vi "Counter.vi"() -> ()   [LabVIEW 2017]
uses:
  <vilib>/addons/database/Connection.llb/DB Tools Open Connec (String).vi
  Global/Global 1.vi
  <vilib>/addons/database/NI_Database_API.lvlib
panel:
  in  "Reset Square":bool
  in  "RECIPE NAME":string
  out "RUNNING LOADED RECIPE":string
  in  "BARCODE RECIPE":string(combo)
  in  "Delete Square":bool
  in  "Save Square":bool
  in  "OK2":bool
  in  "FROM":timestamp format="%<%x>T"
  out "error out":errorcluster
  in  "error in (no error)":errorcluster
  in  "EXIT":bool
  in  "SHIFT":string(combo)
  in  "TO":timestamp format="%<%x>T"
  out "OK":i32
  out "TOTAL":i32
  out "NOK":i32
  # "COUNTER"
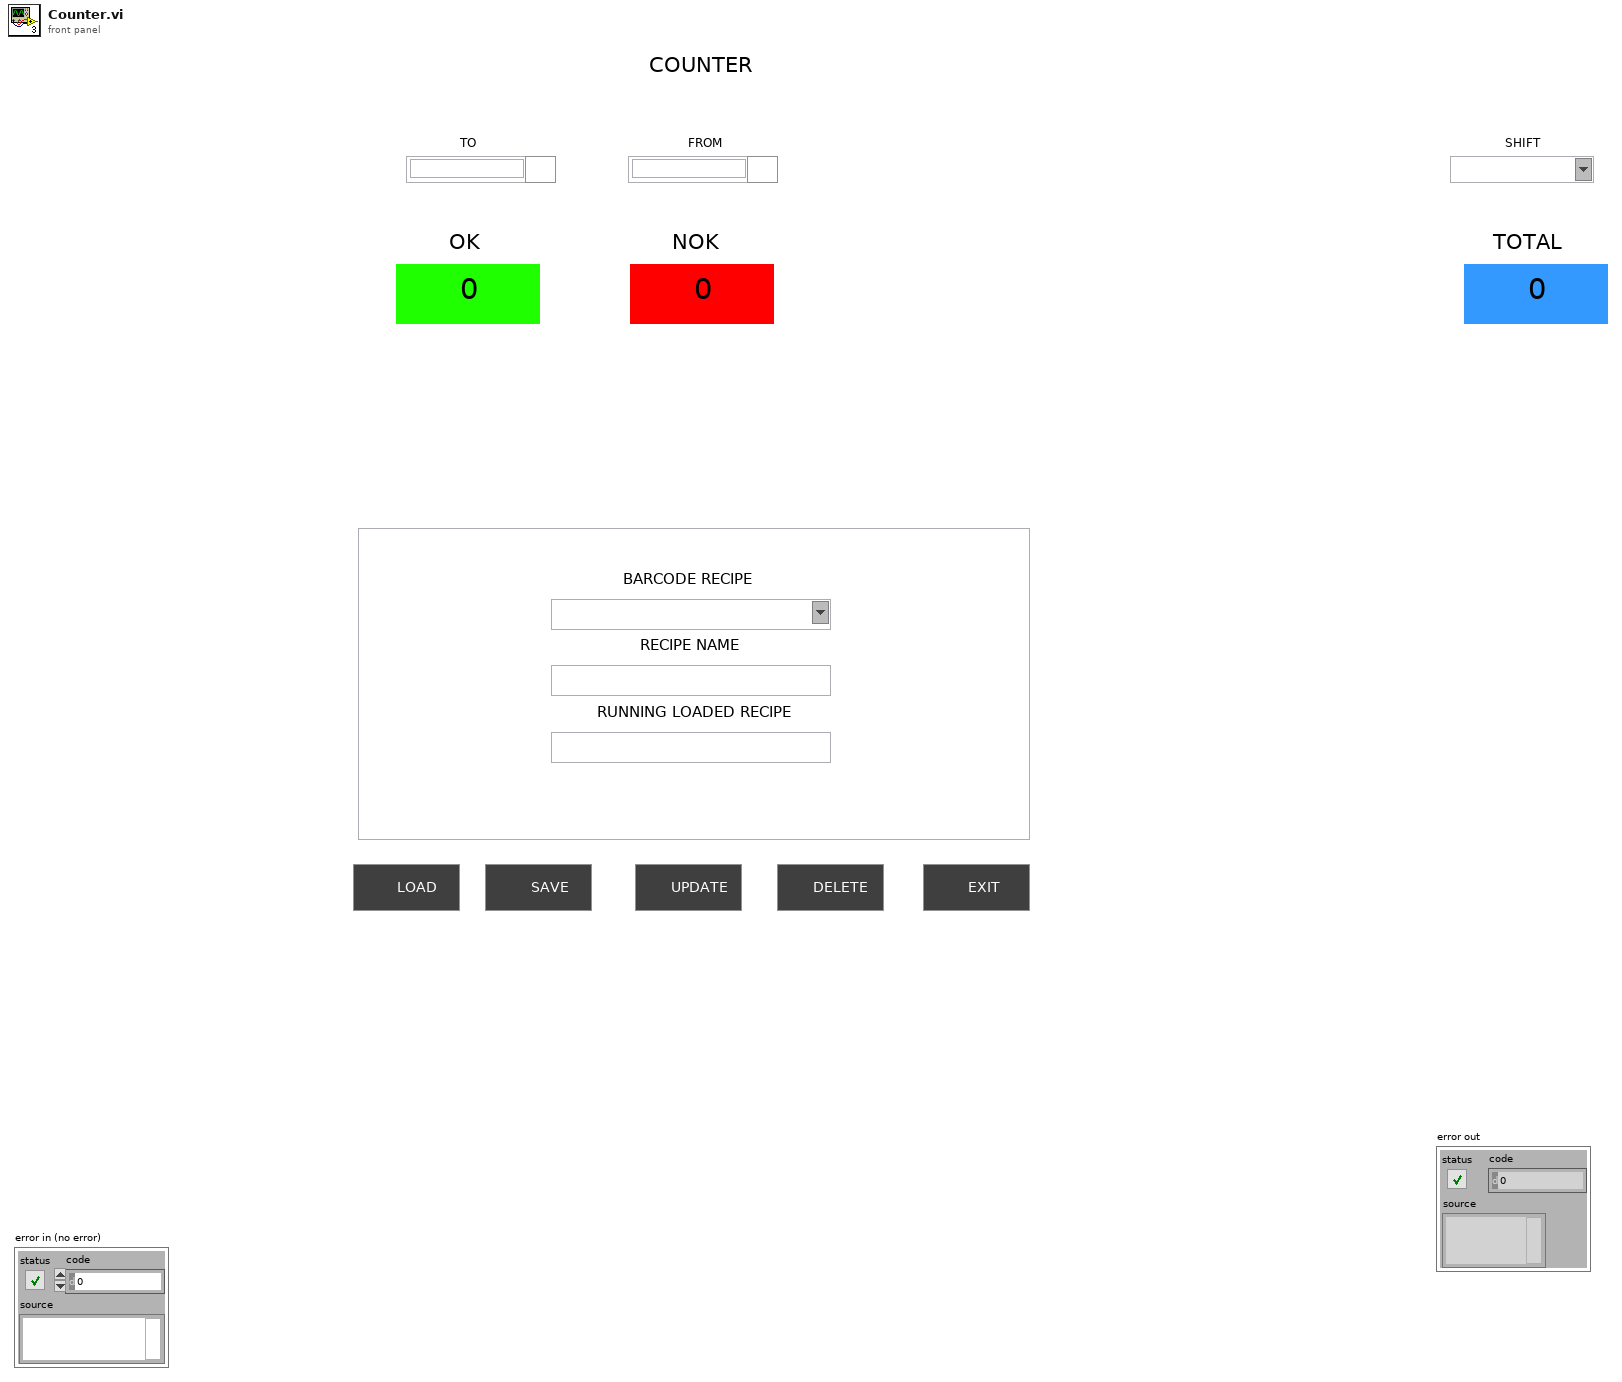
[diagram p1: front panel]
types:
  T1 = typedef "NI_Database_API.lvlib/Conn ObjectReference.ctl" = refnum<k1>
  T2 = cluster{" BARCODE RECIPE":string, "RECIPE NAME":string}
  T3 = enum32{"invalid app kind", "Development System", "Run Time System", "Student Edition", "Embedded LabVIEW", "Evaluation", "Custom"}
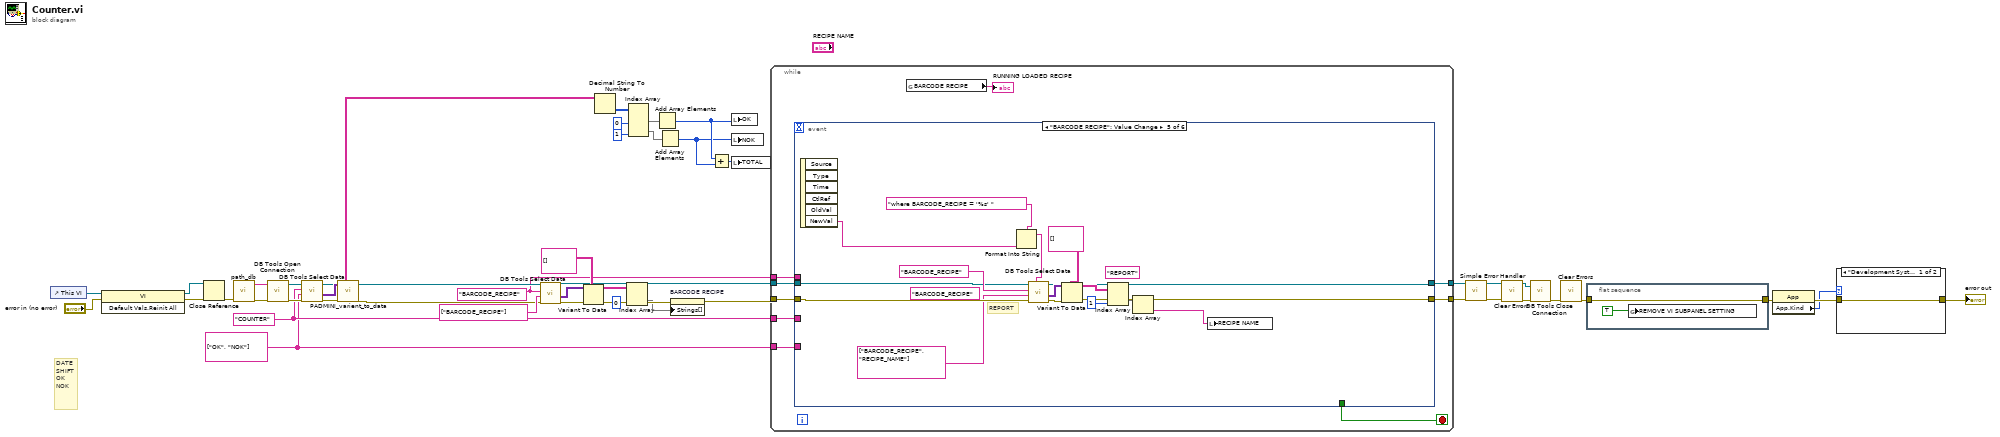
[diagram p0: block diagram]
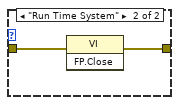
[diagram p2: hidden frame]
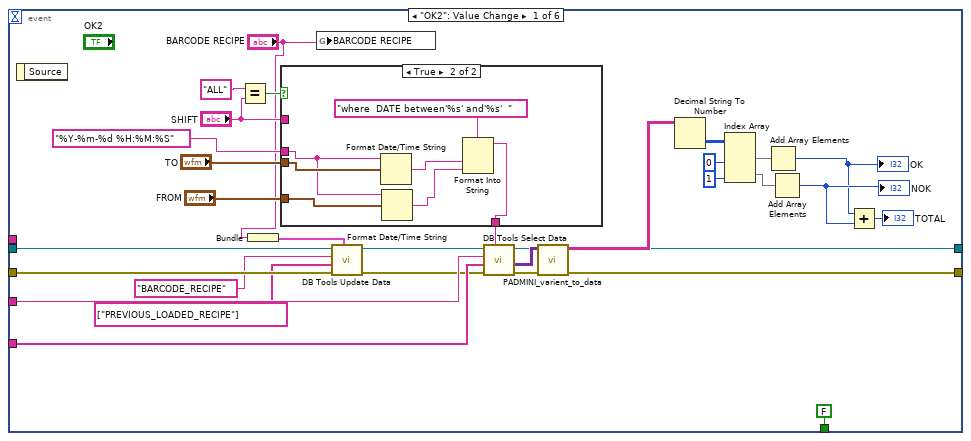
[diagram p3: hidden frame]
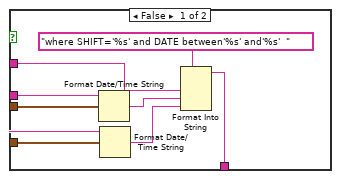
[diagram p4: hidden frame]
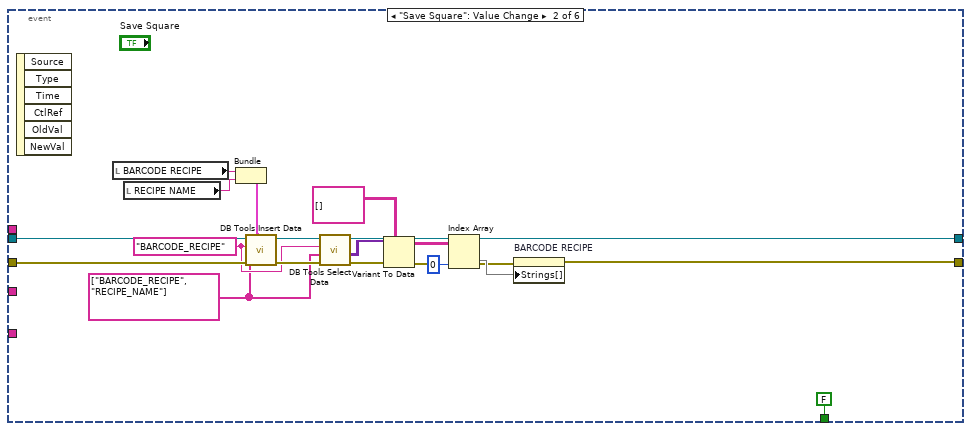
[diagram p5: hidden frame]
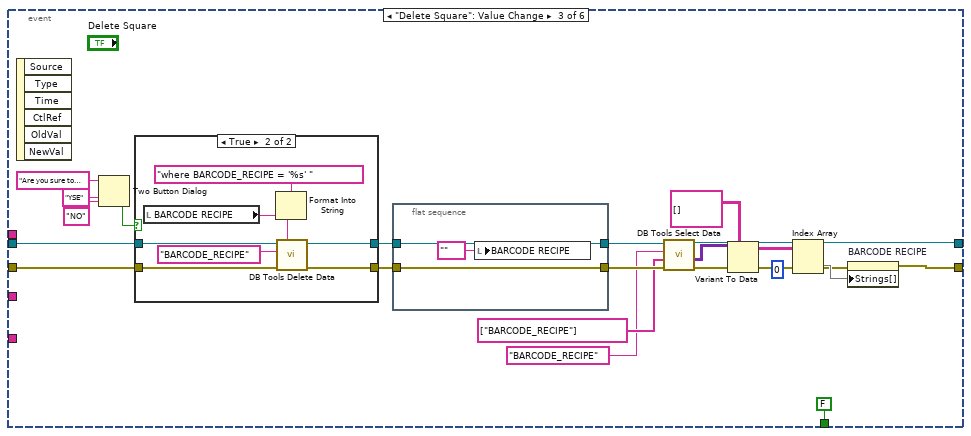
[diagram p6: hidden frame]
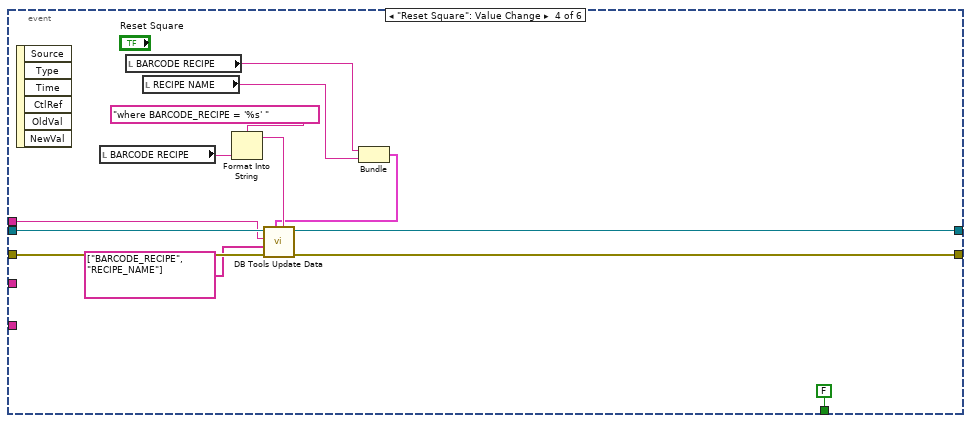
[diagram p8: hidden frame]
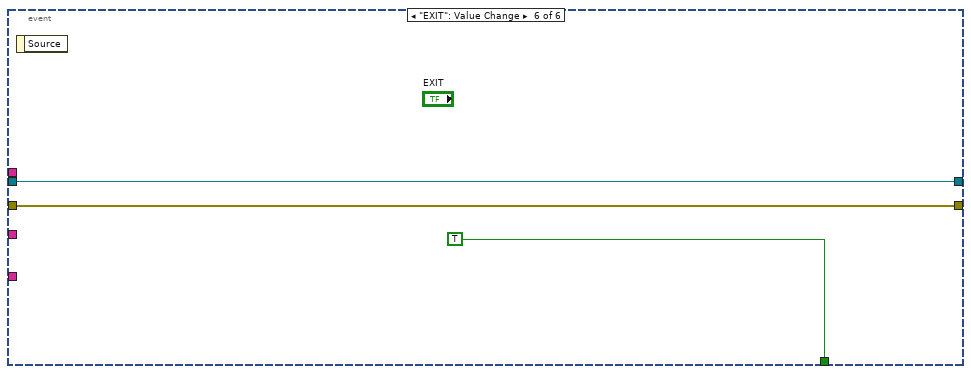
[diagram p9: hidden frame]
diagram:
  w1 = "BARCODE_RECIPE" ("table")
  w14 = string[] ["OK", "NOK"]
  w15 = "COUNTER"
  # "DATE\nSHIFT\nOK\nNOK"
  n1 = control-ref of="This VI"() -> (w43:refnum<vi>)
  n2 = invoke class="VI" method="Default Vals.Reinit All"(reference=w43, error in="error in (no error)") -> (reference out=w41:refnum<vi>, error out=w40:errorcluster)  [unwired: 1 in, 1 out]
  n3 = Close Reference(reference=w41, error in (no error)=w40) -> (error out=w39:errorcluster)
  n4 = call "path_db.vi"("error in"=w39) -> ("error out"=w45:errorcluster, "resulting string"=w44:string)  [unwired: 9 in]
  n5 = call-poly <vilib>:"DB Tools Open Connection.vi"("error in (no error)"=w45, "connection information"=w44) -> ("error out"=w26:errorcluster, "connection reference"=w38:T1)  [unwired: 6 in]
  n6 = call <vilib>:"DB Tools Select Data.vi"("error in (no error)"=w26, "columns"=w14, "table"=w15, "connection reference"=w38) -> ("error out"=w25:errorcluster, "data"=w27:variant[][], "connection reference out"=w4:T1)  [unwired: 2 in]
  n7 = call "PADMINI_varient_to_data.vi"("error in (no error)"=w25, "data"=w27) -> ("error out"=w2:errorcluster, "Array"=w24:string[][])  [unwired: 8 in]
  n8 = call <vilib>:"DB Tools Select Data.vi"("error in (no error)"=w2, "columns"=string[] ["BARCODE_RECIPE"], "table"=w1, "connection reference"=w4) -> ("error out"=w11:errorcluster, "data"=w7:variant[][], "connection reference out"=w5:T1)  [unwired: 2 in]
  n9 = Variant To Data(error in=w11, type=string[][] [], Variant=w7) -> (data=w6:string[][], error out=w13:errorcluster)
  n10 = Decimal String To Number(string=w24) -> (number=w23:i32[][])  [unwired: 2 in, 1 out]
  n11 = Index Array(array=w6, index (col)=0 ("disabled index (col)")) -> (element=w9:string[])  [unwired: 1 in]
  n12 = Index Array(array=w23, index (col) #1=0 ("disabled index (col)"), index (col) #2=1 ("index (col)")) -> (element #1=w20:i32[], element #2=w19:i32[])  [unwired: 2 in]
  n13 = Add Array Elements(numeric array=w20) -> (sum=w18:i32)
  n14 = Add Array Elements(numeric array=w19) -> (sum=w17:i32)
  n15 = property on="BARCODE RECIPE" class="CmbBox"(error in=w13, "Strings[]"=w9) -> (error out=w10:errorcluster)  [unwired: 1 in, 1 out]
  n16 = Add(x=w18, y=w17) -> (x+y=w16:i32)
  n17 = local write "OK"(w18) -> ()
  n18 = local write "NOK"(w17) -> ()
  n19 = local write "TOTAL"(w16) -> ()
  n20 = while {
    tunnel: w10 -> [w53]
    tunnel: w5 -> [w52]
    tunnel: [w51] -> w29
    tunnel: [w50] -> w28
    tunnel: w15 -> [w49]
    tunnel: w14 -> [w48]
    tunnel: w1 -> [w46]
    stop <- w54 stop-if-true
    n21 = event shown="[4] \"BARCODE RECIPE\": Value Change" {
      selector: _ -> [_ _ _ _ _ _]
      dyn-events: _ -> [_ _ _ _ _ _]
      timeout: _ -> [_ _ _ _ _ _]
      tunnel: [FALSE FALSE FALSE FALSE _ TRUE] -> w54
      tunnel: w53 -> [w60 w119 w140 w166 w176 w184]
      tunnel: w52 -> [w62 w118 w141 w167 w177 w185]
      tunnel: [w76 w111 w128 w165 w170 w185] -> w51
      tunnel: [w77 w104 w127 w164 w169 w184] -> w50
      tunnel: w49 -> [w75 _ _ _ _ _]
      tunnel: w48 -> [w74 _ _ _ _ _]
      tunnel: w46 -> [_ _ _ w163 _ _]
      event "OK2": Value Change {
        n22 = event-data() -> ()  [unwired: 1 in, 1 out]
        n23 = Equal?(x="ALL", y="SHIFT") -> (x = y?=w65:bool)
        n24 = Bundle("BARCODE RECIPE"="BARCODE RECIPE") -> (w55:cluster{" BARCODE RECIPE":string})  [unwired: 1 in]
        n25 = case shown="True" w65 {
          tunnel: [w93 w95] -> w70
          tunnel: "SHIFT" -> [w91 _]
          tunnel: "TO" -> [w90 w99]
          tunnel: "FROM" -> [w88 w97]
          tunnel: "%Y-%m-%d %H:%M:%S" ("time format string (%c)") -> [w86 w98]
          frame False {
            n26 = Format Date/Time String(time format string (%c)=w86, seconds (now)=w90) -> (date/time string=w89:string)  [unwired: 1 in]
            n27 = Format Date/Time String(time format string (%c)=w86, seconds (now)=w88) -> (date/time string=w87:string)  [unwired: 1 in]
            n28 = Format Into String(format string="where SHIFT='%s' and DATE between'%s' and'%s'  ", w91, w89, w87) -> (resulting string=w93:string)  [unwired: 2 in, 1 out]
          }
          frame True {
            n29 = Format Date/Time String(time format string (%c)=w98, seconds (now)=w99) -> (date/time string=w100:string)  [unwired: 1 in]
            n30 = Format Date/Time String(time format string (%c)=w98, seconds (now)=w97) -> (date/time string=w96:string)  [unwired: 1 in]
            n31 = Format Into String(format string="where  DATE between'%s' and'%s'  ", w100, w96) -> (resulting string=w95:string)  [unwired: 2 in, 1 out]
          }
        }
        n32 = global write "Global 1.vi" "BARCODE RECIPE"("BARCODE RECIPE") -> ()
        n33 = call <vilib>:"DB Tools Update Data.vi"("data"=w55, "error in (no error)"=w60, "columns"=string[] ["PREVIOUS_LOADED_RECIPE"], "table"="BARCODE_RECIPE", "connection reference"=w62) -> ("error out"=w59:errorcluster, "connection reference out"=w61:T1)  [unwired: 5 in]
        n34 = call <vilib>:"DB Tools Select Data.vi"("condition"=w70, "error in (no error)"=w59, "columns"=w74, "table"=w75, "connection reference"=w61) -> ("error out"=w78:errorcluster, "data"=w85:variant[][], "connection reference out"=w76:T1)  [unwired: 1 in]
        n35 = call "PADMINI_varient_to_data.vi"("error in (no error)"=w78, "data"=w85) -> ("error out"=w77:errorcluster, "Array"=w84:string[][])  [unwired: 8 in]
        n36 = Decimal String To Number(string=w84) -> (number=w83:i32[][])  [unwired: 2 in, 1 out]
        n37 = Index Array(array=w83, index (col) #1=0 ("disabled index (col)"), index (col) #2=1 ("index (col)")) -> (element #1=w80:i32[], element #2=w79:i32[])  [unwired: 2 in]
        n38 = Add Array Elements(numeric array=w80) -> (sum=w71:i32)
        "OK" <- w71
        n39 = Add Array Elements(numeric array=w79) -> (sum=w72:i32)
        "NOK" <- w72
        n40 = Add(x=w71, y=w72) -> (x+y=→"TOTAL":i32)
      }
      event "Save Square": Value Change {
        w102 = string[] ["BARCODE_RECIPE", "RECIPE_NAME"] ("columns")
        w103 = "BARCODE_RECIPE" ("table")
        n41 = event-data() -> ()  [unwired: 1 in, 6 out]
        n42 = local read "BARCODE RECIPE"() -> (w117:string)
        n43 = local read "RECIPE NAME"() -> (w101:string)
        n44 = Bundle("BARCODE RECIPE"=w117, "RECIPE NAME"=w101) -> (w116:T2)  [unwired: 1 in]
        n45 = call <vilib>:"DB Tools Insert Data.vi"("data"=w116, "error in (no error)"=w119, "columns"=w102, "table"=w103, "connection reference"=w118) -> ("error out"=w114:errorcluster, "connection reference out"=w112:T1)  [unwired: 5 in]
        n46 = call <vilib>:"DB Tools Select Data.vi"("error in (no error)"=w114, "columns"=w102, "table"=w103, "connection reference"=w112) -> ("error out"=w113:errorcluster, "data"=w109:variant[][], "connection reference out"=w111:T1)  [unwired: 2 in]
        n47 = Variant To Data(error in=w113, type=string[][] [], Variant=w109) -> (data=w108:string[][], error out=w105:errorcluster)
        n48 = Index Array(array=w108, index (col)=0 ("disabled index (col)")) -> (element=w106:string[])  [unwired: 1 in]
        n49 = property on="BARCODE RECIPE" class="CmbBox"(error in=w105, "Strings[]"=w106) -> (error out=w104:errorcluster)  [unwired: 1 in, 1 out]
      }
      event "Delete Square": Value Change {
        n50 = event-data() -> ()  [unwired: 1 in, 6 out]
        n51 = Two Button Dialog(message="Are you sure to want delete this barcode recipe?", 1:"NO" ("F button name (\"Cancel\")"), 2:"YSE" ("T button name (\"OK\")")) -> (T button?=w121:bool)
        n52 = case shown="True" w121 {
          tunnel: w141 -> [w143 w151]
          tunnel: w140 -> [w142 w150]
          tunnel: [w142 w146] -> w139
          tunnel: [w143 w145] -> w138
          frame False {
          }
          frame True {
            n53 = local read "BARCODE RECIPE"() -> (w148:string)
            n54 = Format Into String(format string="where BARCODE_RECIPE = '%s' ", w148) -> (resulting string=w147:string)  [unwired: 2 in, 1 out]
            n55 = call <vilib>:"DB Tools Delete Data.vi"("condition"=w147, "error in (no error)"=w150, "table"="BARCODE_RECIPE", "connection reference"=w151) -> ("error out"=w146:errorcluster, "connection reference out"=w145:T1)  [unwired: 6 in]
          }
        }
        n56 = flat-sequence {
          tunnel: [w154] -> w129
          tunnel: w139 -> [w154]
          tunnel: [w152] -> w130
          tunnel: w138 -> [w152]
          frame #0 {
            n57 = local write "BARCODE RECIPE"("" ("BARCODE RECIPE")) -> ()
          }
        }
        n58 = call <vilib>:"DB Tools Select Data.vi"("error in (no error)"=w129, "columns"=string[] ["BARCODE_RECIPE"], "table"="BARCODE_RECIPE", "connection reference"=w130) -> ("error out"=w137:errorcluster, "data"=w136:variant[][], "connection reference out"=w128:T1)  [unwired: 2 in]
        n59 = Variant To Data(error in=w137, type=string[][] [], Variant=w136) -> (data=w135:string[][], error out=w133:errorcluster)
        n60 = Index Array(array=w135, index (col)=0 ("disabled index (col)")) -> (element=w134:string[])  [unwired: 1 in]
        n61 = property on="BARCODE RECIPE" class="CmbBox"(error in=w133, "Strings[]"=w134) -> (error out=w127:errorcluster)  [unwired: 1 in, 1 out]
      }
      event "Reset Square": Value Change {
        n62 = event-data() -> ()  [unwired: 1 in, 6 out]
        n63 = local read "BARCODE RECIPE"() -> (w161:string)
        n64 = local read "BARCODE RECIPE"() -> (w158:string)
        n65 = local read "RECIPE NAME"() -> (w157:string)
        n66 = Format Into String(format string="where BARCODE_RECIPE = '%s' ", w161) -> (resulting string=w159:string)  [unwired: 2 in, 1 out]
        n67 = Bundle("BARCODE RECIPE"=w158, "RECIPE NAME"=w157) -> (w156:T2)  [unwired: 1 in]
        n68 = call <vilib>:"DB Tools Update Data.vi"("condition"=w159, "data"=w156, "error in (no error)"=w166, "columns"=string[] ["BARCODE_RECIPE", "RECIPE_NAME"], "table"=w163, "connection reference"=w167) -> ("error out"=w164:errorcluster, "connection reference out"=w165:T1)  [unwired: 4 in]
      }
      event "BARCODE RECIPE": Value Change {
        (unwired) "BARCODE_RECIPE" ("String")
        (unwired) "REPORT"
        # "REPORT"
        n69 = event-data() -> ("NewVal"=w173:string)  [unwired: 1 in, 5 out]
        n70 = Format Into String(format string="where BARCODE_RECIPE = '%s' ", w173) -> (resulting string=w174:string)  [unwired: 2 in, 1 out]
        n71 = call <vilib>:"DB Tools Select Data.vi"("condition"=w174, "error in (no error)"=w176, "columns"=string[] ["BARCODE_RECIPE", "RECIPE_NAME"], "table"="BARCODE_RECIPE", "connection reference"=w177) -> ("error out"=w182:errorcluster, "data"=w181:variant[][], "connection reference out"=w170:T1)  [unwired: 1 in]
        n72 = Variant To Data(error in=w182, type=string[][] [], Variant=w181) -> (data=w180:string[][], error out=w169:errorcluster)
        n73 = Index Array(array=w180, index (col)=1 ("disabled index (col)")) -> (element=w178:string[])  [unwired: 1 in]
        n74 = Index Array(array=w178) -> (element=w168:string)  [unwired: 1 in]
        n75 = local write "RECIPE NAME"(w168) -> ()
      }
      event "EXIT": Value Change {
        n76 = event-data() -> ()  [unwired: 1 in, 1 out]
      }
    }
    n77 = global read "Global 1.vi" "BARCODE RECIPE"() -> (→"RUNNING LOADED RECIPE":string)
  }
  n78 = call <vilib>:"Simple Error Handler.vi"("error in (no error)"=w28) -> ("error out"=w35:errorcluster)  [unwired: 4 in, 4 out]
  n79 = call <vilib>:"Clear Errors.vi"("error in (no error)"=w35) -> ("error out"=w34:errorcluster)  [unwired: 5 in, 1 out]
  n80 = call <vilib>:"DB Tools Close Connection.vi"("error in (no error)"=w34, "connection reference"=w29) -> ("error out"=w37:errorcluster)  [unwired: 5 in]
  n81 = call <vilib>:"Clear Errors.vi"("error in (no error)"=w37) -> ("error out"=w31:errorcluster)  [unwired: 5 in, 1 out]
  n82 = flat-sequence {
    tunnel: w31 -> [w188]
    tunnel: [w188] -> w30
    frame #0 {
      n83 = global write "Global 1.vi" "REMOVE VI SUBPANEL SETTING"(TRUE ("remove_VI")) -> ()
    }
  }
  n84 = property class="App"(error in=w30) -> (error out=w33:errorcluster, "App.Kind"=w32:T3)  [unwired: 1 in, 1 out]
  n85 = case shown="\"Development System\", Default" w32 {
    tunnel: [w189 w191] -> w36
    tunnel: w33 -> [w189 w190]
    frame "Development System", Default {
    }
    frame "Run Time System" {
      n86 = invoke class="VI" method="FP.Close"(error in=w190) -> (error out=w191:errorcluster)  [unwired: 2 in, 2 out]
    }
  }
  "error out" <- w36
